vi "成绩管理.vi"() -> ()   [LabVIEW 2016]
uses:
  <vilib>/express/express arith-compare/Formula/XNode/ExpressFormulaBlockNode.xnode
panel:
  out "及格":bool
  out "成绩等级":string
  out "平均成绩":dbl
  in  "英语":i16 min=0 max=100
  in  "数学":i16 min=0 max=100
  in  "语文":i16 min=0 max=100
  # "学生成绩"
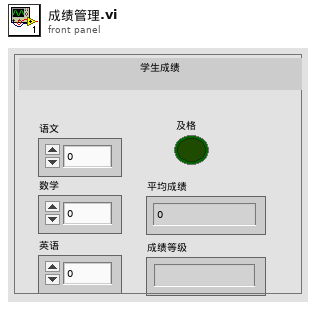
[diagram p1: front panel]
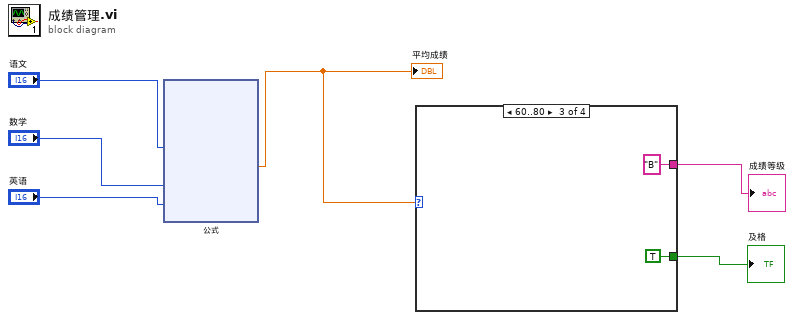
[diagram p0: block diagram]
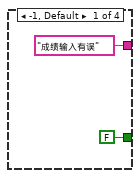
[diagram p2: hidden frame]
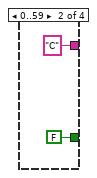
[diagram p3: hidden frame]
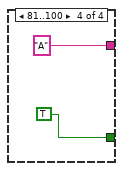
[diagram p4: hidden frame]
diagram:
  n1 = xnode "公式"("语文"="语文", "数学"="数学", "英语"="英语") -> ("结果"=w3:dbl)  [unwired: 1 in, 1 out]
  "平均成绩" <- w3
  n2 = case shown="60..80" w3 {
    tunnel: ["成绩输入有误" ("成绩等级") "C" ("成绩等级") "B" ("成绩等级") "A" ("成绩等级")] -> w2
    tunnel: [FALSE ("及格") FALSE ("及格") TRUE ("及格") TRUE ("及格")] -> w1
    frame -1, Default {
    }
    frame 0..59 {
    }
    frame 60..80 {
    }
    frame 81..100 {
    }
  }
  "成绩等级" <- w2
  "及格" <- w1
